vi "Read configuration.vi"(8 "error in":errorcluster, 11 "dds editor node in":refnum<class "dds editor node.lvclass">) -> (0 "error out":errorcluster, 2 "configuration":refnum<class "NISE_CEF_serializable configuration.lvclass">, 3 "dds editor node out":refnum<class "dds editor node.lvclass">)   [LabVIEW 2020, in "DDS editor node.lvclass"]
uses:
  dds editor node.lvclass
  <vilib>/NI/Configuration Framework/serializable configuration/NISE_CEF_serializable configuration.lvclass
  dds editor node.lvclass/dds editor node.ctl
  module/configuration/dds configuration.lvclass
  C:/Program Files (x86)/National Instruments/LabVIEW 2020/vi.lib/NI/Configuration Framework/serializable configuration/NISE_CEF_serializable configuration.lvclass
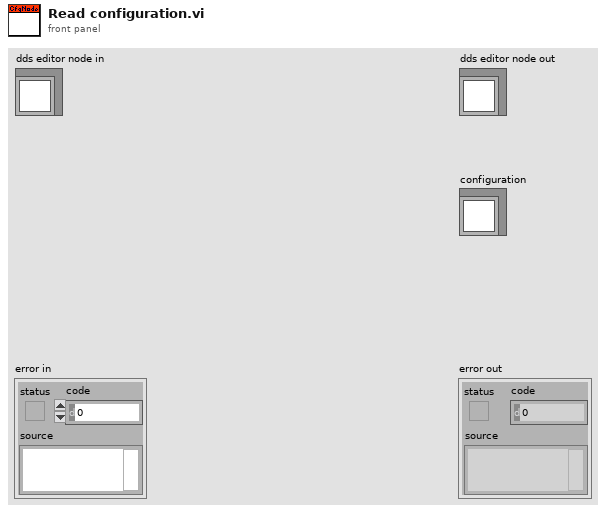
[diagram p1: front panel]
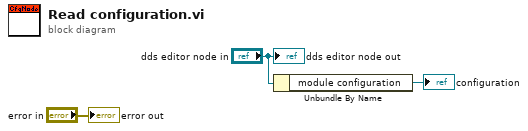
[diagram p0: block diagram]
diagram:
  n1 = Unbundle By Name("dds editor node in") -> ("module configuration"=→"configuration":refnum<class "dds configuration.lvclass">)
  "error out" <- "error in"
  "dds editor node out" <- "dds editor node in"
